vi "Create.vi"(8 "error in (no error)":errorcluster, 11 "EventMessenger in":refnum<class "EventMessenger.lvclass">) -> (0 "error out":errorcluster, 3 "EventMessenger out":refnum<class "EventMessenger.lvclass">)   [LabVIEW 2011, in "Messenging.lvlib" / "EventMessenger.lvclass"]
uses:
  EventMessenger.lvclass
  TextVarientMessage/MSG.lvclass
  EventMessenger.lvclass/EventMessenger.ctl
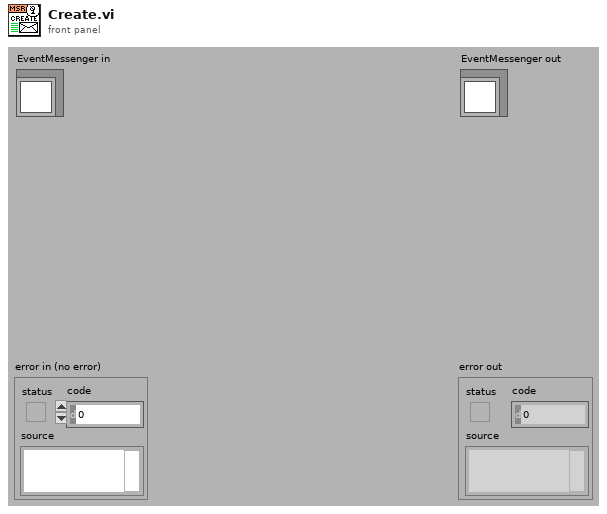
[diagram p1: front panel]
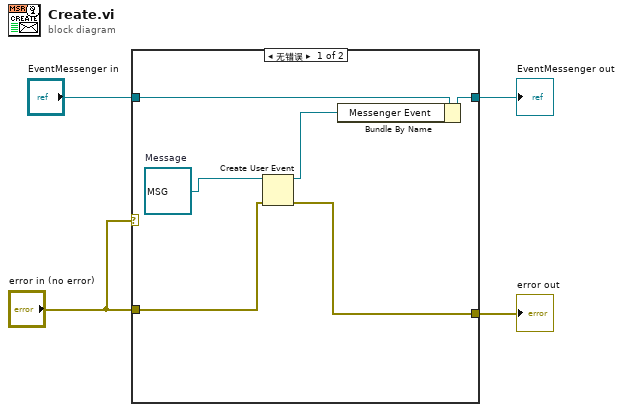
[diagram p0: block diagram]
diagram:
  n1 = case shown="无错误" "error in (no error)" {
    tunnel: "EventMessenger in" -> [w9 w12]
    tunnel: "error in (no error)" -> [w8 w11]
    tunnel: [w7 w11] -> w3
    tunnel: [w6 w12] -> w2
    frame No Error {
      w10 = refnum<class "MSG.lvclass"> refnum  # Message
      n2 = Create User Event(user event datatype=w10, error in=w8) -> (user event=w5:refnum<user-event>, error out=w7:errorcluster)
      n3 = Bundle By Name(cluster=w9, "Messenger Event"=w5) -> (w6:refnum<class "EventMessenger.lvclass">)
    }
    frame Error {
    }
  }
  "error out" <- w3
  "EventMessenger out" <- w2
